vi "TriggerSwitch (SubVI).vi"(0 "data":dynamicdata(waveform), 1 "TRIGGER SW":bool, 3 "Trigger Axis":enum32{"Channel 1", "Channel 2", "Channel 3"}(ring), 5 "Trigger Level":dbl=0.1 format="%#_13g", 9 "Samples to Read":i32, 11 "error in (no error)":errorcluster, 12 "Trigger Slope":enum16{"Falling Edge", "Rising Edge"}(ring)=enum."Rising Edge", 14 "Pre Samples":i32) -> (4 "Data Available":bool, 10 "Section":dynamicdata(waveform), 15 "error out":errorcluster)   [LabVIEW 2018]
uses:
  <vilib>/measure/mamon.llb/Trigger Detection for 1 Channel.vi
  <vilib>/measure/NI_MAPro.lvlib
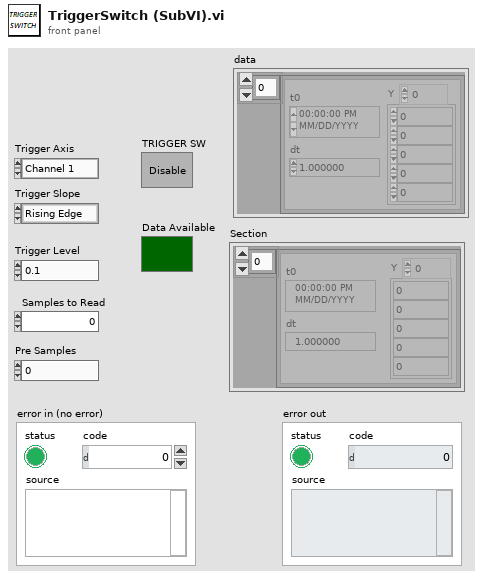
[diagram p1: front panel]
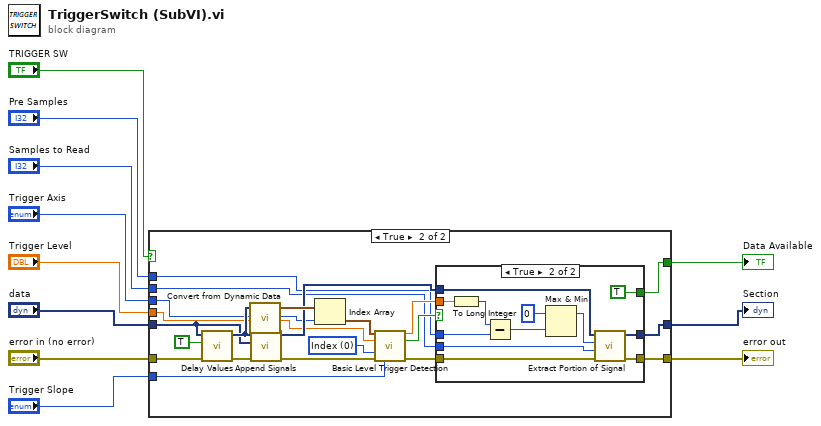
[diagram p0: block diagram]
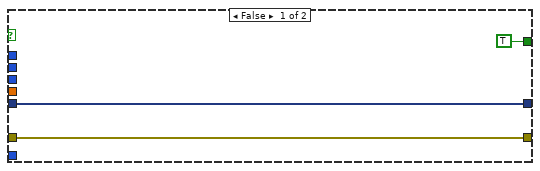
[diagram p2: hidden frame]
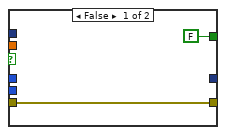
[diagram p3: hidden frame]
diagram:
  n1 = case shown="True" "TRIGGER SW" {
    tunnel: [TRUE ("Data Available") w22] -> w10
    tunnel: "data" -> [w14 w27]
    tunnel: [w14 w20] -> w6
    tunnel: "error in (no error)" -> [w13 w29]
    tunnel: [w13 w21] -> w8
    tunnel: "Samples to Read" -> [_ w19]
    tunnel: "Trigger Axis" -> [_ w18]
    tunnel: "Trigger Slope" -> [_ w17]
    tunnel: "Pre Samples" -> [_ w16]
    tunnel: "Trigger Level" -> [_ w15]
    frame False {
    }
    frame True {
      w33 = u16 0 items=["Index", "Time"] ("location mode")
      n2 = call "Delay Values"("error in (no error)"=w29, "Enable"=TRUE, "Signals"=w27) -> ("error out"=w26:errorcluster, "Delayed Signals"=w28:dynamicdata)  [unwired: 7 in]
      n3 = call "Convert from Dynamic Data"("Dynamic Data Type"=w28) -> ("Array of Waveform"=w35:waveform(dbl)[])  [unwired: 3 in]
      n4 = call "Append Signals"("error in (no error)"=w26, "Input Signal B"=w27, "Input Signal A"=w28) -> ("error out"=w25:errorcluster, "Appended Signals"=w23:dynamicdata)  [unwired: 7 in]
      n5 = Index Array(array=w35, index=w18) -> (element=w34:waveform(dbl))
      n6 = call-poly <vilib>:"Basic Level Trigger Detection.vi"("signal in"=w34, "level"=w15, "location mode"=w33, "error in (no error)"=w25, "trigger slope"=w17) -> ("trigger location"=w31:dbl, "trigger detected?"=w32:bool, "error out"=w24:errorcluster)  [unwired: 8 in]
      n7 = case shown="True" w32 {
        tunnel: w31 -> [_ w48]
        tunnel: w24 -> [w36 w49]
        tunnel: w23 -> [_ w43]
        tunnel: [FALSE ("Enable") TRUE ("Enable")] -> w22
        tunnel: [w36 w46] -> w21
        tunnel: [_ w44] -> w20
        tunnel: w16 -> [_ w41]
        tunnel: w19 -> [_ w38]
        frame False {
        }
        frame True {
          n8 = To Long Integer(number=w48) -> (32bit integer=w47:i32)
          n9 = Subtract(x=w47, y=w41) -> (x-y=w42:i32)
          n10 = Max & Min(x=0, y=w42) -> (max(x,y)=w39:i32)  [unwired: 1 out]
          n11 = call "Extract Portion of Signal"("error in (no error)"=w49, "Samples"=w38, "Begin Sample"=w39, "Signals"=w43) -> ("error out"=w46:errorcluster, "Section"=w44:dynamicdata)  [unwired: 6 in]
        }
      }
    }
  }
  "Data Available" <- w10
  "error out" <- w8
  "Section" <- w6
